vi "niRFSysCalReader Fetch Source Offset.vi"(8 "error in":errorcluster, 9 "Desired Output Power (dBm)":dbl, 10 "Frequency (Hz)":dbl, 11 "niRFSysCalReader Handle":T1) -> (0 "error out":errorcluster, 2 "Source Offset (dB)":dbl, 3 "niRFSysCalReader Handle out":T1)   [LabVIEW 2016, in "niRFSysCalReader.lvlib"]
doc: "Returns the source offset for the specified frequency and desired output power. The source offset is the path loss of the external path that is connected to the signal generator's output port.\n\n<b>Note:</b> To acheive the desired output power, make the signal generator's output power attribute equal to the specified <b>Desired Output Power (dBm)</b>'s value and make the signal generator's external gain attribute equal to the result of negating the returned <b>Source Offset (dB)</b>'s value.\ni.e.\nSignal Generator's Output Power = Desired Output Power \nSignal Generator's External Gain = -1 * Source Offset"
uses:
  niRFSysCalReader.lvlib
  _INCLUDES/niRFSysCalReader Handle.ctl
  _INCLUDES/niRFSysCalReader Core States.ctl
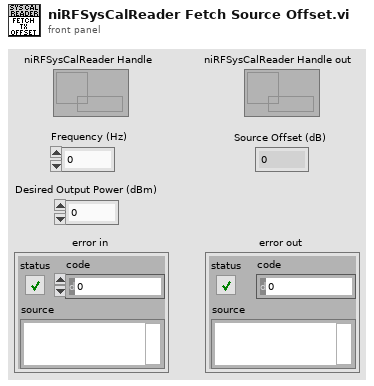
[diagram p1: front panel]
types:
  T1 = typedef "niRFSysCalReader.lvlib/niRFSysCalReader Handle.ctl" = refnum<data-value>
  T2 = typedef "niRFSysCalReader.lvlib/niRFSysCalReader Core States.ctl" = enum16{"Initialize", "Interpolator State", "Add Pathloss", "Get Pathloss", "Remove Pathloss", "Close"}
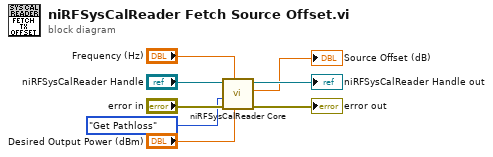
[diagram p0: block diagram]
diagram:
  n1 = call "niRFSysCalReader Core.vi"("Power (dBm)"="Desired Output Power (dBm)", "Frequency (Hz)"="Frequency (Hz)", "error in"="error in", "niRFSysCalReader State"=niRFSysCalReader_Core_States."Get Pathloss" ("Cal Storage"), "niRFSysCalReader Handle"="niRFSysCalReader Handle") -> ("error out"=→"error out":errorcluster, "Pathloss (dB)"=→"Source Offset (dB)":dbl, "niRFSysCalReader Handle out"=→"niRFSysCalReader Handle out":T1)  [unwired: 4 in]
